vi "GaGe_ChannelConfigAll.vi"(3 "Channel (0)":u32 step=1, 4 "V scale":T2 {"Coupling" items=["DC 1 MOhm", "AC 1 MOhm", "DC 50 Ohm", "AC 50 OHM"]; "Offset" format="%.2f"}, 5 "Handle Cluster":T1) -> (2 "Handle Cluster Out":T1)   [LabVIEW 2022 SP3]
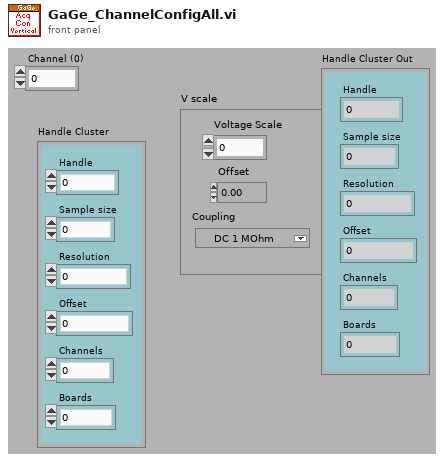
[diagram p1: front panel]
types:
  T1 = cluster{"Handle":u32, "Sample size":u32, "Resolution":i32, "Offset":i32, "Channels":u32, "Boards":u32}
  T2 = cluster{"Voltage Scale":dbl, "Offset":dbl, "Coupling":u16}
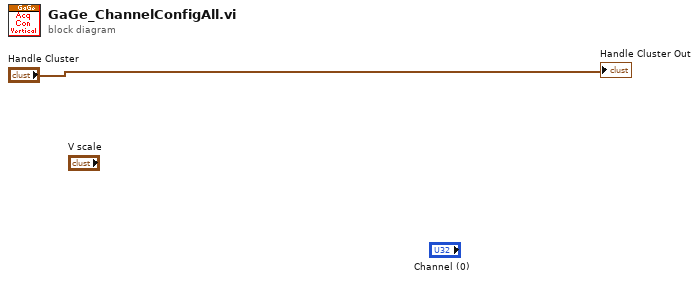
[diagram p0: block diagram]
diagram:
  "Handle Cluster Out" <- "Handle Cluster"
